vi "DWF MSO Configure Analog Edge Trigger.vi"(0 "Instrument Handle In":u32, 1 "Trigger Hysteresis":dbl=0.01, 5 "Trigger Source":string, 7 "Trigger Slope":i32(ring) items=["Rising", "Falling", "Either"], 9 "Trigger Level":dbl, 11 "Error In":errorcluster caption="Error In (no error)", 12 "Trigger Instance":i32(ring) items=["A", "B"]) -> (4 "Instrument Handle Out":u32, 15 "Error Out":errorcluster)   [LabVIEW 2015, in "DigilentWF.lvlib"]
doc: "Configures a trigger to activate on the specified source when the analog edge reaches the specified levels."
uses:
  <vilib>/DigilentWF/DigilentWF.lvlib
  dwf.dll
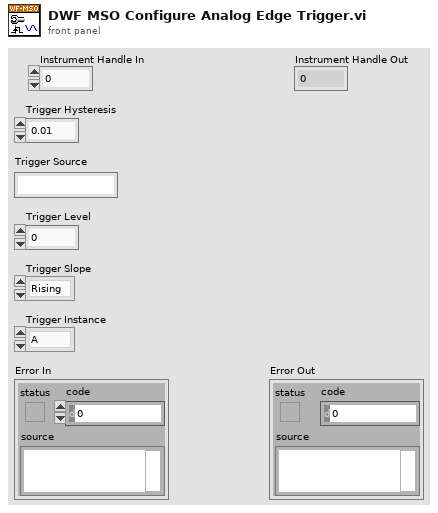
[diagram p1: front panel]
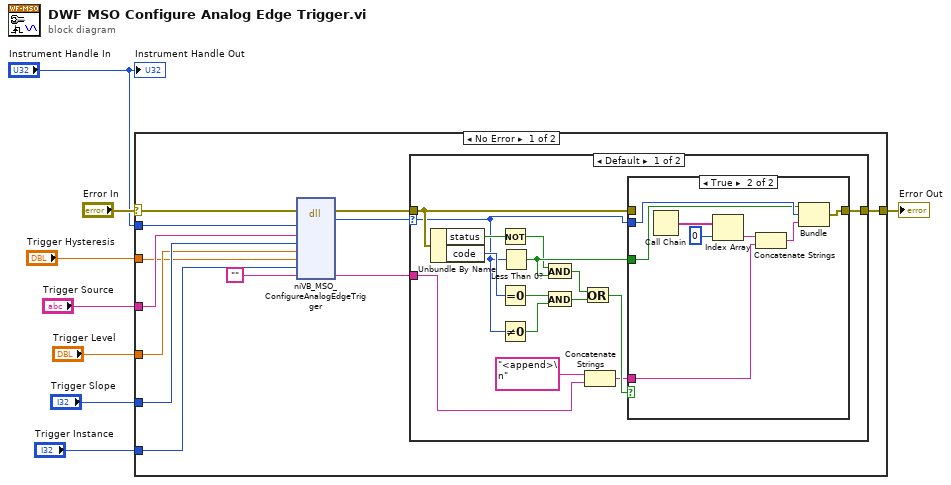
[diagram p0: block diagram]
diagram:
  n1 = case "outter_case" shown="No Error" "Error In" {
    selector: "Error In" -> [w19 w46]
    tunnel: [w20 w46] -> w7
    tunnel: "Instrument Handle In" -> [w16 _]
    tunnel: "Trigger Hysteresis" -> [w12 _]
    tunnel: "Trigger Source" -> [w15 _]
    tunnel: "Trigger Level" -> [w13 _]
    tunnel: "Trigger Slope" -> [w14 _]
    tunnel: "Trigger Instance" -> [w11 _]
    frame No Error {
      n2 = dll-call lib="dwf.*" fn="niVB_MSO_ConfigureAnalogEdgeTrigger"(error in=w19, "instrumentHandle"=w16, "triggerSource"=w15, "triggerSlope"=w14, "triggerLevel"=w13, "triggerHysteresis"=w12, "triggerInstance"=w11, "szError"="") -> (error out=w18:errorcluster, "return type"=w17:i32, "szError"=w9:string)  [unwired: 8 in, 1 out]
      n3 = case "inner_case" shown="Default" w17 {
        selector: w17 -> [w25 _]
        tunnel: w18 -> [w26 w45]
        tunnel: [w22 w45] -> w20
        tunnel: w9 -> [w21 _]
        frame Default {
          n4 = Unbundle By Name(w26) -> ("status"=w30:bool, "code"=w34:i32)
          n5 = Not(x=w30) -> (.not. x?=w33:bool)
          n6 = Equal To 0?(x=w34) -> (x = 0?=w29:bool)
          n7 = Not Equal To 0?(x=w25) -> (x != 0?=w32:bool)
          n8 = Less Than 0?(x=w25) -> (x < 0?=w35:bool)
          n9 = And(x=w33, y=w35) -> (x .and. y?=w31:bool)
          n10 = And(x=w29, y=w32) -> (x .and. y?=w28:bool)
          n11 = Or(x=w31, y=w28) -> (x .or. y?=w27:bool)
          n12 = Concatenate Strings("<append>\n" ("string"), w21) -> (w24:string)
          n13 = case shown="True" w27 {
            tunnel: [w36 w43] -> w22
            tunnel: w25 -> [_ w42]
            tunnel: w35 -> [_ w41]
            tunnel: w26 -> [w36 _]
            tunnel: w24 -> [_ w37]
            frame False {
            }
            frame True {
              n14 = Call Chain() -> (call chain=w40:string[])
              n15 = Index Array(array=w40, index=0) -> (element=w39:string)
              n16 = Concatenate Strings(w39, w37) -> (w44:string)
              n17 = Bundle(w41, "return type"=w42, w44) -> (w43:cluster{bool, "return type":i32, string})  [unwired: 1 out]
            }
          }
        }
        frame 0 {
        }
      }
    }
    frame Error {
    }
  }
  "Error Out" <- w7
  "Instrument Handle Out" <- "Instrument Handle In"
